vi "Read Type Override.vi"(8 "error in (no error)":errorcluster, 11 "CIF_Fifo_Raw_Multi in":refnum<class "CIF_Fifo_Raw_Multi.lvclass">) -> (0 "error out":errorcluster, 2 "Type Override":string, 3 "CIF_Fifo_Raw_Multi out":refnum<class "CIF_Fifo_Raw_Multi.lvclass">)   [LabVIEW 2021, in "CIF_Fifo_Raw_Multi.lvclass"]
uses:
  CIF_Fifo_Raw_Multi.lvclass
  CIF_Fifo_Raw_Multi.lvclass/CIF_Fifo_Raw_Multi.ctl
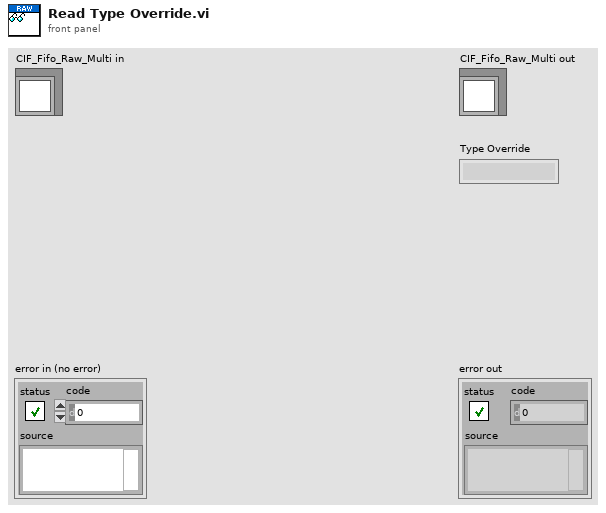
[diagram p1: front panel]
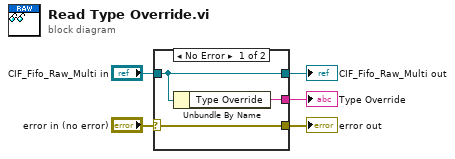
[diagram p0: block diagram]
diagram:
  n1 = case shown="No Error" "error in (no error)" {
    selector: "error in (no error)" -> [w8 w9]
    tunnel: [w8 w9] -> w4
    tunnel: [w7 w10] -> w2
    tunnel: "CIF_Fifo_Raw_Multi in" -> [w7 w10]
    tunnel: [w6 _] -> w1
    frame No Error {
      n2 = Unbundle By Name(w7) -> ("Type Override"=w6:string)
    }
    frame Error {
    }
  }
  "error out" <- w4
  "CIF_Fifo_Raw_Multi out" <- w2
  "Type Override" <- w1
